vi "Check Settings.vi"(8 "error in (no error)":errorcluster, 10 "Iterator Settings in":T1={"Prepare timeout (ms)"=200, "Iterate timeout (ms)"=50, "Conclude timeout (ms)"=200, "Iterate period (ms)"=200, "Number of iterations"=5, "Time before stop (ms)"=5, "Active Stop Conditions"={"Number of Iterations"=FALSE, "Time Elapsed"=FALSE, "Iteration Result"=FALSE}, "Prepare Msg"=refnum, "Iterate Msg"=refnum, "Conclude Msg"=refnum, "Iterations End Report"=refnum, "Message Priority (Normal)"=enum."Normal"}, 11 "Iterator Actor in":refnum<class "Iterator Actor.lvclass">) -> (0 "error out":errorcluster, 2 "Iterator Settings out":T1={"Prepare timeout (ms)"=200, "Iterate timeout (ms)"=50, "Conclude timeout (ms)"=200, "Iterate period (ms)"=200, "Number of iterations"=5, "Time before stop (ms)"=5, "Active Stop Conditions"={"Number of Iterations"=FALSE, "Time Elapsed"=FALSE, "Iteration Result"=FALSE}, "Prepare Msg"=refnum, "Iterate Msg"=refnum, "Conclude Msg"=refnum, "Iterations End Report"=refnum, "Message Priority (Normal)"=enum."Normal"}, 3 "Iterator Actor out":refnum<class "Iterator Actor.lvclass">)   [LabVIEW 2023, in "Iterator Actor.lvlib" / "Iterator Actor.lvclass"]
doc: "Checks the input settings of the iterator. \nReturns an error with a description if something is wrong."
uses:
  Iterator Actor.lvclass
  Abstract Iterator Actor/Iterator Settings.ctl
  Abstract Iterator Actor Messages/Iterator Report Iterations End Msg/Iterator Report Iterations End Msg.lvclass
  <vilib>/ActorFramework/Message/Message.lvclass
  Abstract Iterator Actor/Active Stop Conditions.ctl
  <vilib>/ActorFramework/Message Enqueuer/Message Priority.ctl
  Iterator Actor Messages/Iterator Reply Msg/Iterator Reply Msg.lvclass
  <vilib>/Utility/error.llb/Error Cluster From Error Code.vi
  Abstract Iterator Actor/Abstract Iterator Actor.lvclass
  <vilib>/ErrorRing/Error Ring.xnode
  Iterator Actor.lvclass/Iterator Actor.ctl
  <vilib>/ActorFramework/Message Enqueuer/Message Enqueuer.lvclass
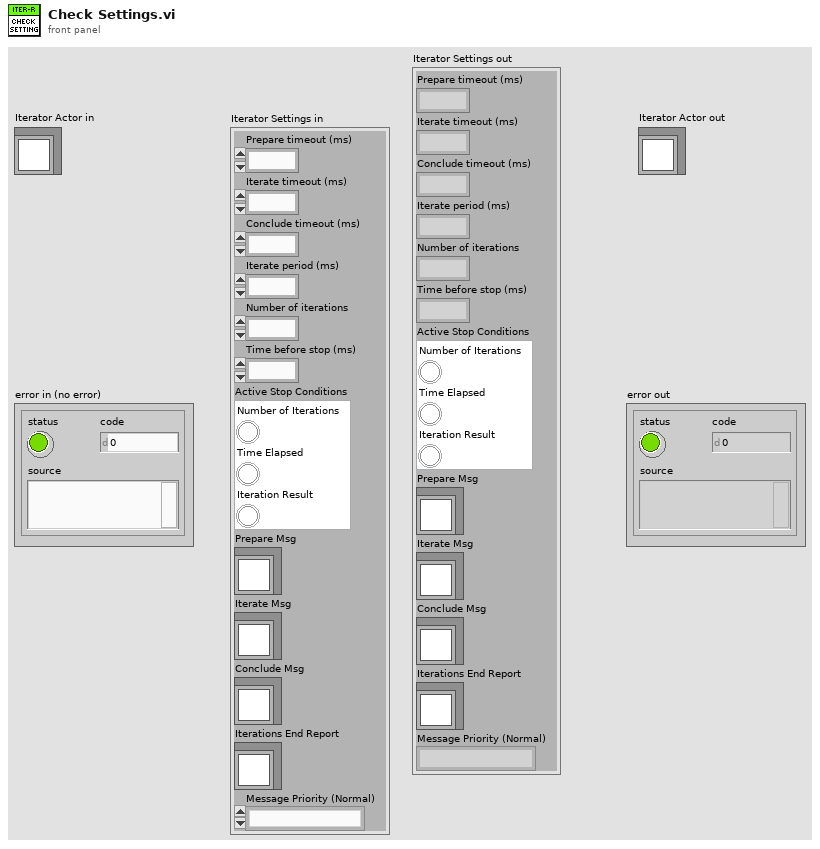
[diagram p1: front panel]
types:
  T1 = typedef "Iterator Actor.lvlib/Abstract Iterator Actor.lvclass/Iterator Settings.ctl" = cluster{"Prepare timeout (ms)":i32, "Iterate timeout (ms)":i32, "Conclude timeout (ms)":i32, "Iterate period (ms)":i32, "Number of iterations":i32, "Time before stop (ms)":i32, "Active Stop Conditions":T2, "Prepare Msg":refnum<class "Message.lvclass">, "Iterate Msg":refnum<class "Message.lvclass">, "Conclude Msg":refnum<class "Message.lvclass">, "Iterations End Report":refnum<class "Iterator Report Iterations End Msg.lvclass">, "Message Priority (Normal)":T3}
  T2 = typedef "Iterator Actor.lvlib/Abstract Iterator Actor.lvclass/Active Stop Conditions.ctl" = cluster{"Number of Iterations":bool, "Time Elapsed":bool, "Iteration Result":bool}
  T3 = typedef "Actor Framework.lvlib/Message Enqueuer.lvclass/Message Priority.ctl" = enum16{"Low", "Normal", "High"}
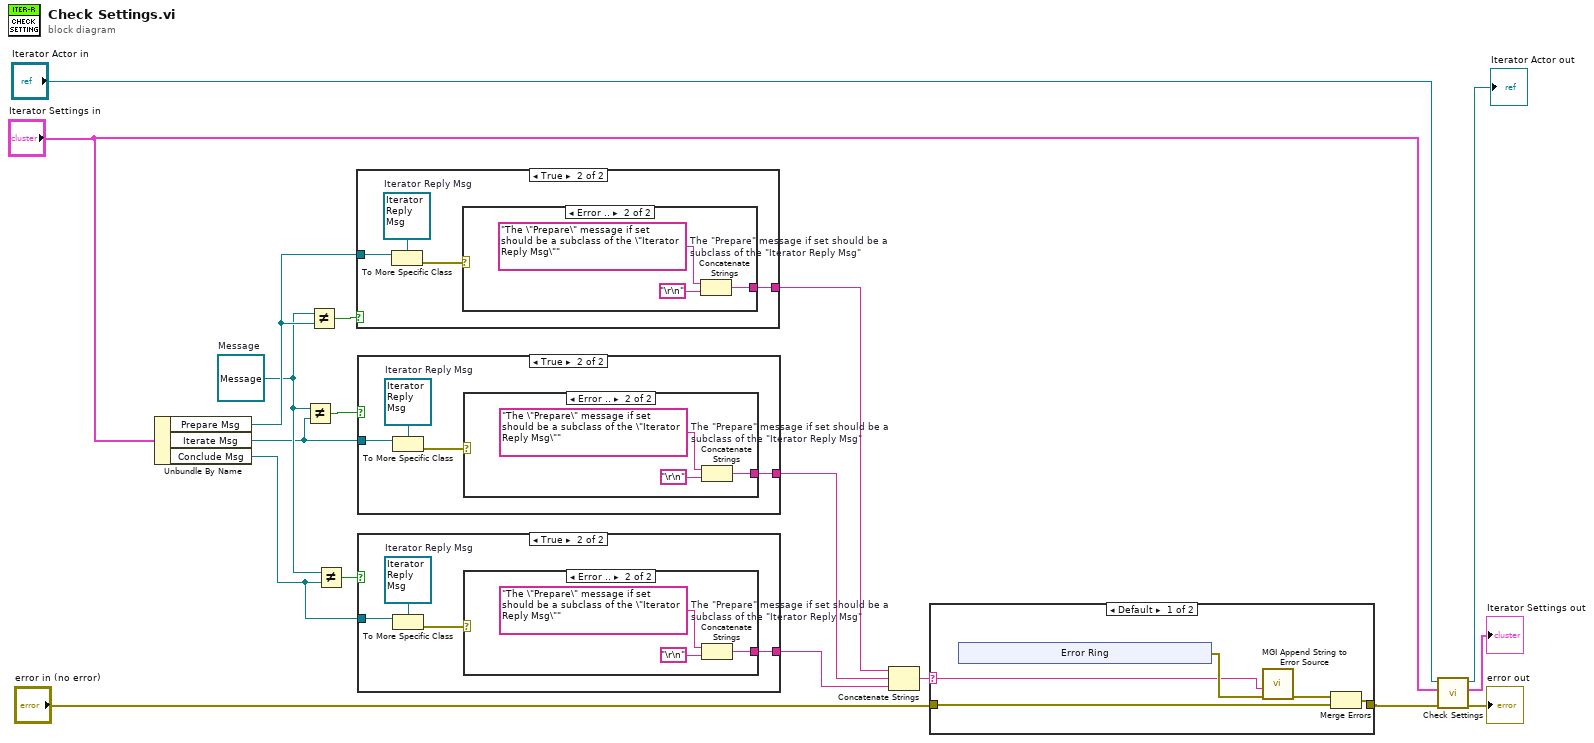
[diagram p0: block diagram]
diagram:
  w12 = refnum<class "Message.lvclass"> refnum  # Message
  n1 = Unbundle By Name("Iterator Settings in") -> ("Prepare Msg"=w13:refnum<class "Message.lvclass">, "Iterate Msg"=w11:refnum<class "Message.lvclass">, "Conclude Msg"=w8:refnum<class "Message.lvclass">)
  n2 = Not Equal?(x=w12, y=w11) -> (x != y?=w10:bool)
  n3 = Not Equal?(x=w12, y=w13) -> (x != y?=w14:bool)
  n4 = Not Equal?(x=w12, y=w8) -> (x != y?=w9:bool)
  n5 = case shown="True" w14 {
    tunnel: w13 -> [_ w22]
    tunnel: [_ w19] -> w7
    frame False {
    }
    frame True {
      w21 = refnum<class "Iterator Reply Msg.lvclass"> refnum  # Iterator Reply Msg
      n6 = To More Specific Class(target class=w21, reference=w22) -> (error out=w20:errorcluster)  [unwired: 1 in, 1 out]
      n7 = case shown="Error .." w20 {
        tunnel: [_ w23] -> w19
        frame No Error {
        }
        frame Error {
          w25 = "The \"Prepare\" message if set should be a subclass of the \"Iterator Reply Msg\""  # The "Prepare" message if set should be a subclass of the "Iterator Reply Msg"
          n8 = Concatenate Strings(w25, "\r\n") -> (w23:string)
        }
      }
    }
  }
  n9 = case shown="True" w10 {
    tunnel: w11 -> [_ w29]
    tunnel: [_ w26] -> w6
    frame False {
    }
    frame True {
      w28 = refnum<class "Iterator Reply Msg.lvclass"> refnum  # Iterator Reply Msg
      n10 = To More Specific Class(target class=w28, reference=w29) -> (error out=w27:errorcluster)  [unwired: 1 in, 1 out]
      n11 = case shown="Error .." w27 {
        tunnel: [_ w30] -> w26
        frame No Error {
        }
        frame Error {
          w32 = "The \"Prepare\" message if set should be a subclass of the \"Iterator Reply Msg\""  # The "Prepare" message if set should be a subclass of the "Iterator Reply Msg"
          n12 = Concatenate Strings(w32, "\r\n") -> (w30:string)
        }
      }
    }
  }
  n13 = case shown="True" w9 {
    tunnel: w8 -> [_ w36]
    tunnel: [_ w33] -> w5
    frame False {
    }
    frame True {
      w35 = refnum<class "Iterator Reply Msg.lvclass"> refnum  # Iterator Reply Msg
      n14 = To More Specific Class(target class=w35, reference=w36) -> (error out=w34:errorcluster)  [unwired: 1 in, 1 out]
      n15 = case shown="Error .." w34 {
        tunnel: [_ w37] -> w33
        frame No Error {
        }
        frame Error {
          w39 = "The \"Prepare\" message if set should be a subclass of the \"Iterator Reply Msg\""  # The "Prepare" message if set should be a subclass of the "Iterator Reply Msg"
          n16 = Concatenate Strings(w39, "\r\n") -> (w37:string)
        }
      }
    }
  }
  n17 = Concatenate Strings(w7, w6, w5) -> (w2:string)
  n18 = case shown="Default" w2 {
    selector: w2 -> [w40 _]
    tunnel: "error in (no error)" -> [w44 w49]
    tunnel: [w43 w49] -> w1
    frame Default {
      n19 = xnode "Error Ring"() -> ("error out"=w42:errorcluster)
      n20 = call <userlib>:"MGI Append String to Error Source.vi"("Error In"=w42, "String to Append"=w40) -> ("Error Out"=w41:errorcluster)  [unwired: 9 in]
      n21 = Merge Errors(w41, w44) -> (w43:errorcluster)
    }
    frame "" {
    }
  }
  n22 = call-parent "Check Settings.vi"("error in (no error)"=w1, "Iterator Settings in"="Iterator Settings in", "Abstract Iterator Actor in"="Iterator Actor in") -> ("error out"=→"error out":errorcluster, "Iterator Settings out"=→"Iterator Settings out":T1, "Abstract Iterator Actor out"=→"Iterator Actor out":refnum<class "Iterator Actor.lvclass">)  [unwired: 6 in]
